vi "AuxGlobals.vi"() -> ()   [LabVIEW 2020]
panel:
  in  "FeedDemand":dbl
  in  "ShootDemand":dbl
  in  "BeltDemand":dbl
  in  "ShootButton":i64
  in  "RevButton":i64
  out "Intake UP":bool
  in  "IntakeSpeedDemand":dbl
  in  "BeltSpeedDemand":dbl
  in  "FeederSpeedDemand":dbl
  in  "FeederEncoderDistance":dbl
  in  "ShooterMotorOutput":dbl
  in  "ShooterRPM":dbl
  in  "ShooterSpeedDemand":dbl
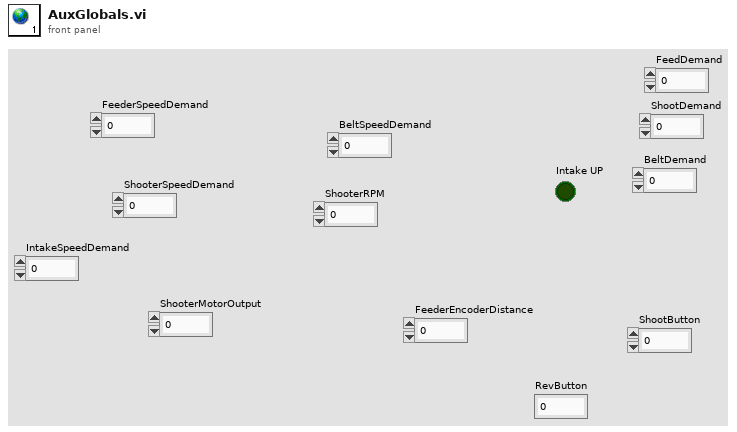
[diagram p1: front panel]
diagram:
